vi "SVPO Power in Band (Complex) (1 Ch).vi"(0 "complex spectrum":T7={"complex spectrum response"={"f0"=0.0, "df"=1.0, "complex spectrum"=[]}, "spectrum info"={"channel name"="", "description"="", "x-axis units"=0, "spectral info"={"spectrum type"=enum."Power [Magnitude^2]", "linear/dB"=enum."linear", "window"=0, "window size"=0, "FFT size"=0}, "engineering units"=0, "custom label"="", "dB reference [EU]"=0.0, "peak units"=enum."rms", "weighting filter"=0, "spectral density?"=FALSE, "unit label"="", "spectrum skewed?"=FALSE, "complimentary spectrum units"=enum."none"}} {"spectrum info"."x-axis units" items=["Time (s)"=0, "Frequency-CB (Hz)"=1, "Frequency-CPB (Hz)"=1248, "Frequency-Arbitrary (Hz)"=2357, "Quefrency (s)"=2, "Revolutions (rev)"=3, "Order"=4, "Speed (RPM)"=11, "Speed (rad/s)"=21, "Index"=65535]; "spectrum info"."weighting filter" items=["Linear", "A-weighting", "B-weighting", "C-weighting", "ITU-R 468-4", "Dolby", "CCITT", "C-message", "Wb", "Wc", "Wd", "We", "Wf", "Wh", "Wj", "Wk", "Wm", "AES17 20 kHz lowpass", "AES17 40 kHz lowpass", "AES17 20 kHz highpass", "AES17 40 kHz highpass"]; "spectrum info"."dB reference [EU]" format="%.2f"; "spectrum info"."engineering units" items=["custom..."=0, "V"=1, "A"=21, "C"=30, "pC"=31, "s"=32, "-"=29, "Pa"=2, "N"=20, "g"=3, "m/s^2"=4, "m/s"=5, "m"=6, "mm/s"=12, "mm"=13, "micron/s"=14, "micron"=15, "in/s^2"=7, "in/s"=8, "in"=9, "mil/s"=10, "mil"=11, "rad/s^2"=16, "rad/s"=17, "rad"=18, "deg/s^2"=26, "deg/s"=27, "deg"=28, "RPM"=22, "cycle/s^2"=23, "Hz"=24, "cycle"=25, "strain"=19]; "spectrum info"."spectral info"."window" items=["None "=0, "Hanning"=1, "Hamming"=2, "Blackman-Harris"=3, "Exact Blackman"=4, "Blackman"=5, "Flat Top"=6, "4 Term B-Harris "=7, "7 Term B-Harris"=8, "Low Sidelobe"=9, "Force - Exponential"=10, "Gaussian"=62]; "complex spectrum response"."complex spectrum" format="%.2f"; "complex spectrum response"."df" format="%.2f"; "complex spectrum response"."f0" format="%.2f"}, 1 "range":cluster{"start":dbl, "stop":dbl}={"start"=-1.0, "stop"=-1.0} {"stop" format="%.2f"; "start" format="%.2f"}) -> (14 "power in band [EU^2 rms]":dbl=nan format="%.2f")   [LabVIEW 2017]
doc: "Computes the aggregate power of a linear-scale power spectrum within the specified frequency <B>range</B> of the input spectrum. Use this VI on embedded targets that have limited computational resources. Wire data to the <B>spectrum [EU^2 rms]</B> input to determine the polymorphic instance to use or manually select the instance."
uses:
  <vilib>/addons/_NISVFA/_Shared subVIs/Controls/svc_Spectrum Info.ctl
  <vilib>/addons/_NISVFA/_Shared subVIs/Controls/svc_X-Axis Units.ctl
  <vilib>/addons/_NISVFA/_Shared subVIs/Controls/svc_Spectrum Type.ctl
  <vilib>/addons/_NISVFA/_Shared subVIs/Controls/svc_Engineering Units Text Ring.ctl
  <vilib>/addons/_NISVFA/_Shared subVIs/Controls/svc_Weighting Filter Text Ring.ctl
  <vilib>/addons/_NISVFA/_Shared subVIs/Controls/svc_Complimentary Spectrum Units.ctl
  <vilib>/Analysis/BLAS.llb/dznrm2 - Vector 2-Norm (CDB).vi
  <vilib>/Analysis/NI_AALBLAS.lvlib
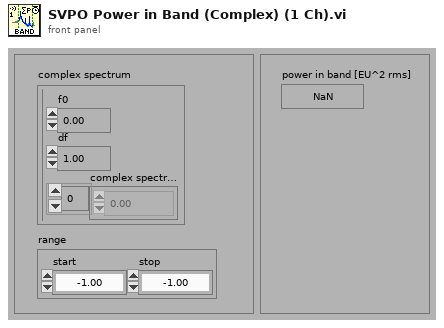
[diagram p1: front panel]
types:
  T1 = typedef "svc_Spectrum Info.ctl" = cluster{"channel name":string, "description":string, "x-axis units":T2, "spectral info":cluster{"spectrum type":T3, "linear/dB":enum16{"linear", "dB"}, "window":u16, "window size":i32, "FFT size":i32}, "engineering units":T4, "custom label":string, "dB reference [EU]":dbl, "peak units":enum16{"rms", "peak", "peak-peak"}, "weighting filter":T5, "spectral density?":bool, "unit label":string, "spectrum skewed?":bool, "complimentary spectrum units":T6}
  T2 = typedef "svc_X-Axis Units.ctl" = u16
  T3 = typedef "svc_Spectrum Type.ctl" = enum16{"FFT Spectrum [complex]", "Amplitude [Magnitude]", "Power [Magnitude^2]", "Cross Spectrum [complex]", "Frequency Response [Complex]"}
  T4 = typedef "svc_Engineering Units Text Ring.ctl" = u16
  T5 = typedef "svc_Weighting Filter Text Ring.ctl" = u16
  T6 = typedef "svc_Complimentary Spectrum Units.ctl" = enum16{"none", "radians", "degrees", "cycles", "imaginary"}
  T7 = cluster{"complex spectrum response":cluster{"f0":dbl, "df":dbl, "complex spectrum":cdb[]}, "spectrum info":T1}
  T8 = typedef "NI_AALPro.lvlib/windowTd.ctl" = u32
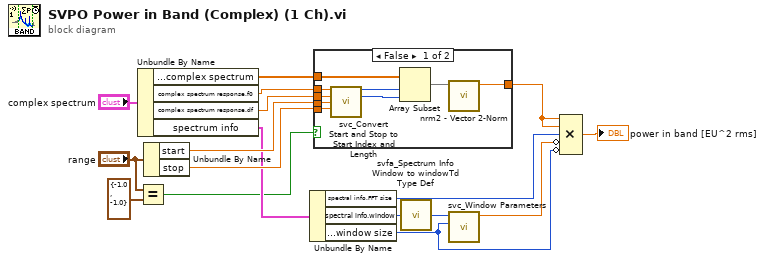
[diagram p0: block diagram]
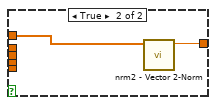
[diagram p2: hidden frame]
diagram:
  n1 = Unbundle By Name("complex spectrum") -> ("complex spectrum response.complex spectrum"=w11:cdb[], "complex spectrum response.f0"=w13:dbl, "complex spectrum response.df"=w7:dbl, "spectrum info"=w6:T1)
  n2 = Equal?(x="range", y=cluster{"start":dbl, "stop":dbl} {"start"=-1.0, "stop"=-1.0}) -> (x = y?=w3:bool)
  n3 = Unbundle By Name("range") -> ("start"=w9:dbl, "stop"=w10:dbl)
  n4 = Unbundle By Name(w6) -> ("spectral info.FFT size"=w12:i32, "spectral info.window"=w16:u16, "spectral info.window size"=w15:i32)
  n5 = case shown="False" w3 {
    tunnel: w13 -> [w26 _]
    tunnel: w11 -> [w20 w28]
    tunnel: w10 -> [w25 _]
    tunnel: w9 -> [w24 _]
    tunnel: w7 -> [w23 _]
    tunnel: [w22 w27] -> w2
    frame False {
      n6 = call <vilib>:"svc_Convert Start and Stop to Start Index and Length.vi"("f0"=w26, "df"=w23, "start frequency"=w24, "stop frequency"=w25) -> ("start index"=w19:i32, "band length"=w18:i32)  [unwired: 8 in, 2 out]
      n7 = Array Subset(array=w20, index=w19, length=w18) -> (w21:cdb[])
      n8 = call-poly <vilib>:"nrm2 - Vector 2-Norm.vi"("x"=w21) -> ("dznrm2"=w22:dbl)  [unwired: 9 in, 1 out]
    }
    frame True {
      n9 = call-poly <vilib>:"nrm2 - Vector 2-Norm.vi"("x"=w28) -> ("dznrm2"=w27:dbl)  [unwired: 9 in, 1 out]
    }
  }
  n10 = call <vilib>:"svfa_Spectrum Info Window to windowTd Type Def.vi"("window"=w16) -> ("window"=w1:T8)  [unwired: 4 in]
  n11 = call <vilib>:"svc_Window Parameters.vi"("window size"=w15, "window"=w1) -> ("ENBW"=w8:dbl)  [unwired: 6 in, 3 out]
  n12 = Compound Arithmetic op=MULTIPLY(w2, w2, w12, invert w8, invert w15) -> (→"power in band [EU^2 rms]":dbl)
